vi "Host-FIXParser-SendData.vi"(8 "error in\n(no error)":errorcluster, 10 "FPGA VI Reference In":T1, 11 "Byte Stream\nFile in":refnum<file>) -> (0 "error out":errorcluster, 2 "data":u8[](array[numeric]) format="%.0x", 3 "FPGA VI Reference Out":T1)   [LabVIEW 2020]
uses:
  FIXParser-TestHarness-Typedef.ctl
  <vilib>/rvi/interface/RandomDataEmulation/nirviRandomDataDMAMethods.vi
  <vilib>/rvi/interface/nirviMethod/nirviMethod.xnode
  Fpga/Tests/Fpga-FIXParser-TestHarness.vi
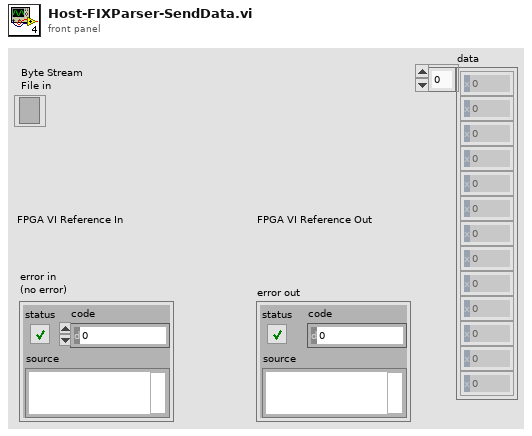
[diagram p1: front panel]
types:
  T1 = typedef "FIXParser-TestHarness-Typedef.ctl" = refnum<k20>
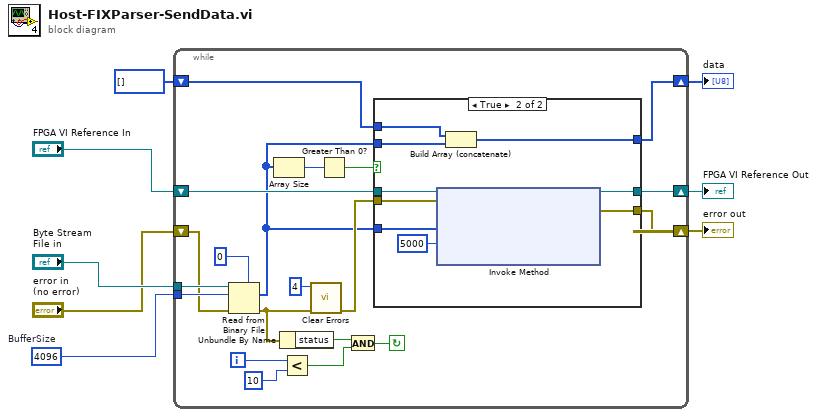
[diagram p0: block diagram]
diagram:
  w7 = 4096  # BufferSize
  n1 = while {
    tunnel: "Byte Stream\nFile in" -> [w28]
    tunnel: w7 -> [w27]
    shift-right: [w20] -> w1
    shift-left: "FPGA VI Reference In" -> [w21]
    shift-right: [w19] -> w3
    shift-left: "error in\n(no error)" -> [w17]
    shift-right: [w11] -> w5
    shift-left: u8[] [] -> [w10]
    i -> [w25]
    stop <- w26 continue-if-true
    n2 = Read from Binary File(5:u8 0 ("data type"), 8:w17, 10:w27, 11:w28) -> (0:w16:errorcluster, 2:w9:u8[])  [unwired: 2 in, 2 out]
    n3 = Array Size(array=w9) -> (size(s)=w15:i32)
    n4 = Unbundle By Name(w16) -> ("status"=w22:bool)
    n5 = Less?(x=w25, y=10) -> (x < y?=w23:bool)
    n6 = call <vilib>:"Clear Errors.vi"("error in (no error)"=w16, "specific error code to clear (0: all)"=4) -> ("error out"=w13:errorcluster)  [unwired: 4 in, 1 out]
    n7 = Greater Than 0?(x=w15) -> (x > 0?=w14:bool)
    n8 = And(x=w22, y=w23) -> (x .and. y?=w26:bool)
    n9 = case shown="True" w14 {
      tunnel: w21 -> [w31 w40]
      tunnel: [w31 w39] -> w20
      tunnel: [w30 w38] -> w19
      tunnel: w13 -> [w30 w36]
      tunnel: w9 -> [_ w32]
      tunnel: [w29 w35] -> w11
      tunnel: w10 -> [w29 w34]
      tunnel: w9 -> [_ w33]
      frame False {
      }
      frame True {
        n10 = xnode "Invoke Method"("FPGA VI Reference In"=w40, "error in"=w36, "Data"=w32, "Timeout (ms)"=5000) -> ("FPGA VI Reference Out"=w39:T1, "error out"=w38:errorcluster)  [unwired: 1 out]
        n11 = Build Array (concatenate)(w34, w33) -> (w35:u8[])
      }
    }
  }
  "error out" <- w3
  "data" <- w5
  "FPGA VI Reference Out" <- w1
